vi "write TBM configuration.vi"(8 "error in":errorcluster, 10 "configuration":refnum<class "TBM configuration.lvclass">, 11 "CVT editor node in":refnum<class "TEC editor node.lvclass">) -> (0 "error out":errorcluster, 3 "CVT editor node out":refnum<class "TEC editor node.lvclass">)   [LabVIEW 2013, in "TEC editor node.lvclass"]
uses:
  TEC editor node.lvclass
  <vilib>/NI/Tag Bus Module Framework/root configuration/TBM configuration.lvclass
  module/configuration/TEC configuration.lvclass
  TEC editor node.lvclass/TEC editor node.ctl
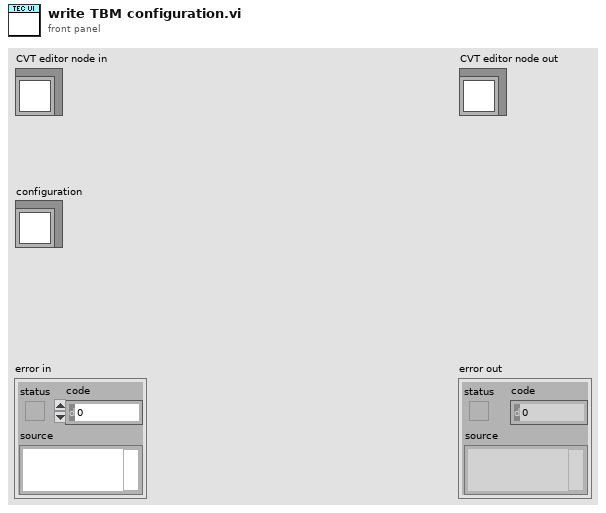
[diagram p1: front panel]
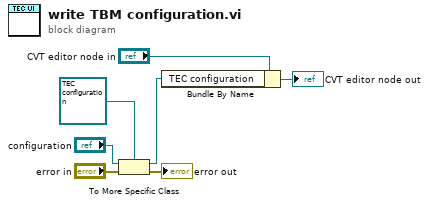
[diagram p0: block diagram]
diagram:
  n1 = To More Specific Class(target class=refnum<class "TEC configuration.lvclass"> refnum ("CVT configuration"), reference="configuration", error in="error in") -> (specific class reference=w1:refnum<class "TEC configuration.lvclass">, error out=→"error out":errorcluster)
  n2 = Bundle By Name(cluster="CVT editor node in", "TEC configuration"=w1) -> (→"CVT editor node out":refnum<class "TEC editor node.lvclass">)
